vi "DigitalGroup_Get Signal Number.vi"(8 "error in":errorcluster, 9 "Recording Cluster":T1) -> (0 "error out":errorcluster, 2 "Num of Signals":u32)   [LabVIEW 2020]
uses:
  <vilib>/express/express signal manip/DigitalDataGroupingXNode/DigitalGroup_Recording Cluster.ctl
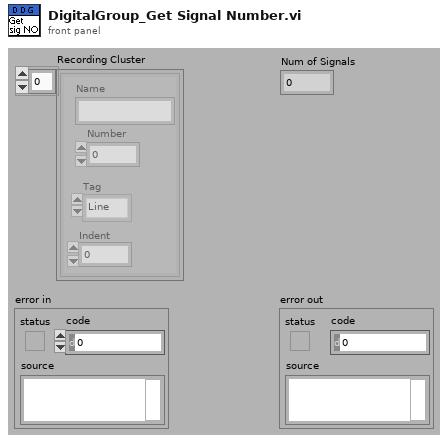
[diagram p1: front panel]
types:
  T1 = typedef "DigitalGroup_Recording Cluster.ctl" = cluster{"Name":string, "Number":u32, "Indent":u32, "Tag":enum16{"Line", "Opened Bus", "Closed Bus"}}[]
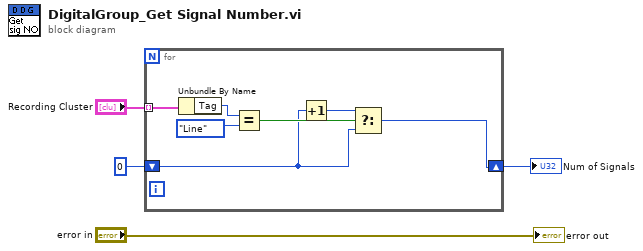
[diagram p0: block diagram]
diagram:
  n1 = for {
    tunnel: "Recording Cluster" -> [w9] mode=indexing
    shift-right: [w10] -> w2
    shift-left: 0 ("disabled index (col)") -> [w6]
    n2 = Unbundle By Name(w9) -> ("Tag"=w8:enum16{"Line", "Opened Bus", "Closed Bus"})
    n3 = Equal?(x=w8, y=enum16{"Line", "Opened Bus", "Closed Bus"}."Line") -> (x = y?=w11:bool)
    n4 = Increment(x=w6) -> (x+1=w7:i32)
    n5 = Select(t=w7, s=w11, f=w6) -> (s? t:f=w10:i32)
  }
  "Num of Signals" <- w2
  "error out" <- "error in"
